vi "Add Test Suite XML Tag.vi"(8 "error in (no error)":errorcluster, 10 "Suite Results":T1, 11 "Reports.lvlib:XML Report.lvclass":refnum<class "XML Report.lvclass">) -> (0 "error out":errorcluster, 3 "output cluster":refnum<class "XML Report.lvclass">)   [LabVIEW 2020, in "XML Report.lvclass"]
doc: "Add a new element to an existing DOM document."
uses:
  XML Report.lvclass
  Suite Result.ctl
  XML Report.lvclass/XML Report.ctl
  <resource>/objmgr/DOMUserDefRef.rc
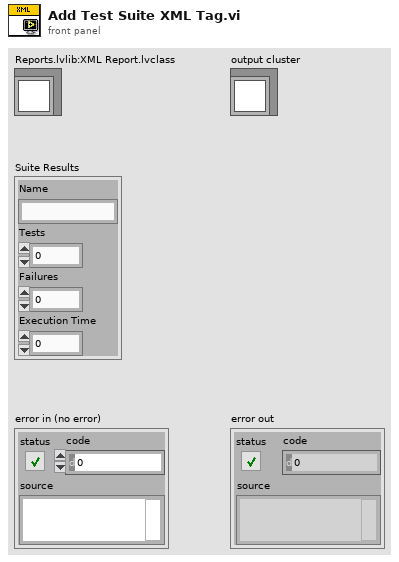
[diagram p1: front panel]
types:
  T1 = typedef "XML Report.lvclass/Suite Result.ctl" = cluster{"Name":string, "Tests":i32, "Failures":i32, "Execution Time":dbl}
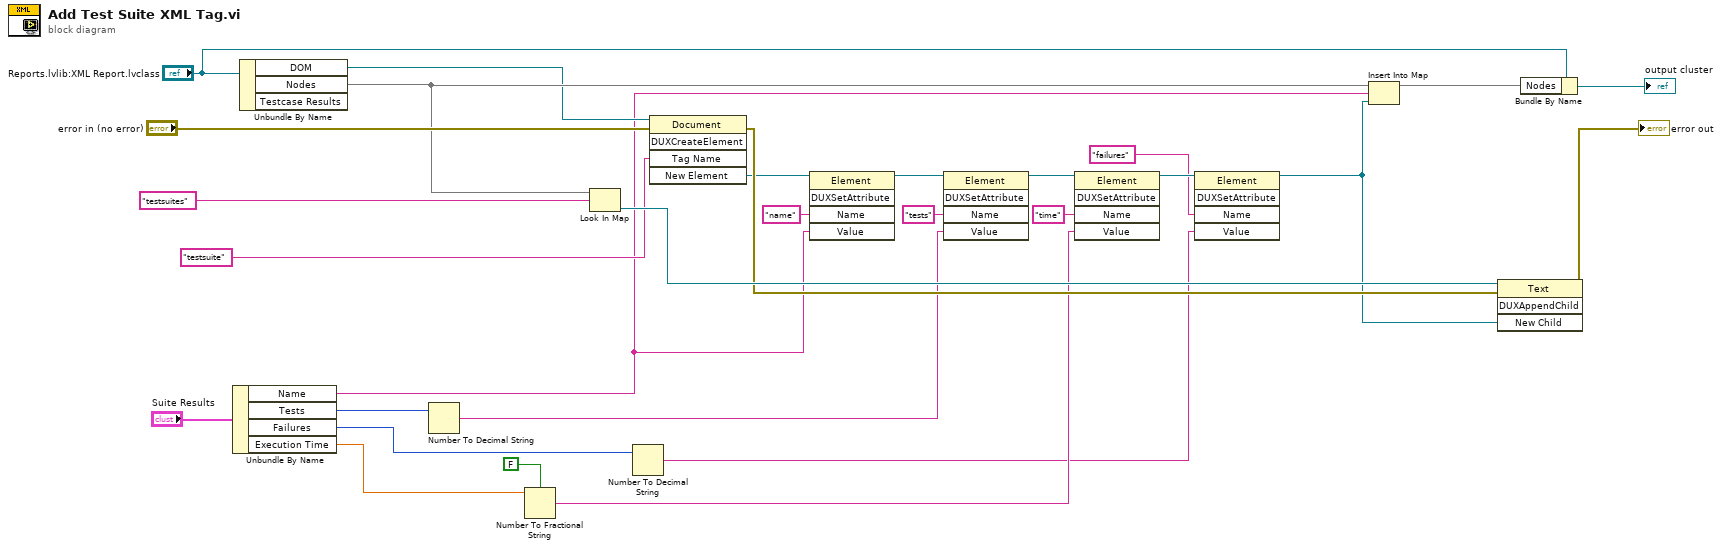
[diagram p0: block diagram]
diagram:
  n1 = Unbundle By Name("Suite Results") -> ("Name"=w15:string, "Tests"=w12:i32, "Failures"=w2:i32, "Execution Time"=w8:dbl)
  n2 = Unbundle By Name("Reports.lvlib:XML Report.lvclass") -> ("DOM"=w21:refnum<k20>, "Nodes"=w26:map{string, refnum<k20>})  [unwired: 1 out]
  n3 = Number To Decimal String(number=w12) -> (decimal integer string=w11:string)  [unwired: 1 in]
  n4 = Number To Fractional String(use system decimal point (T)=FALSE, number=w8) -> (F-format string=w7:string)  [unwired: 2 in]
  n5 = Look In Map(map=w26, key="testsuites" ("Suite Name")) -> (value=w27:refnum<k20>)  [unwired: 1 in, 1 out]
  n6 = Number To Decimal String(number=w2) -> (decimal integer string=w1:string)  [unwired: 1 in]
  n7 = invoke class="Document" method="DUXCreateElement"(reference=w21, error in="error in (no error)", "Tag Name"="testsuite") -> (error out=w22:errorcluster, "New Element"=w18:refnum<k20>)  [unwired: 2 in, 3 out]
  n8 = invoke class="Element" method="DUXSetAttribute"(reference=w18, "Name"="name", "Value"=w15) -> (reference out=w14:refnum<k20>)  [unwired: 2 in, 4 out]
  n9 = invoke class="Element" method="DUXSetAttribute"(reference=w14, "Name"="tests", "Value"=w11) -> (reference out=w10:refnum<k20>)  [unwired: 2 in, 4 out]
  n10 = invoke class="Element" method="DUXSetAttribute"(reference=w10, "Name"="time", "Value"=w7) -> (reference out=w5:refnum<k20>)  [unwired: 2 in, 4 out]
  n11 = invoke class="Element" method="DUXSetAttribute"(reference=w5, "Name"="failures", "Value"=w1) -> (reference out=w4:refnum<k20>)  [unwired: 2 in, 4 out]
  n12 = Insert Into Map(map in=w26, key=w15, value=w4) -> (map out=w24:map{string, refnum<k20>})  [unwired: 2 out]
  n13 = invoke class="Text" method="DUXAppendChild"(reference=w27, error in=w22, "New Child"=w4) -> (error out=→"error out":errorcluster)  [unwired: 1 in, 3 out]
  n14 = Bundle By Name(cluster="Reports.lvlib:XML Report.lvclass", "Nodes"=w24) -> (→"output cluster":refnum<class "XML Report.lvclass">)
